vi "PH_BL-Master.PC _getVacPressuress.vi"(0 "i ref in":refnum<vi>, 2 "Channel Name":string="N/A", 3 "Value":dbl, 5 "error in (no error)":errorcluster) -> (14 "i ref out":refnum<vi>, 19 "error out":errorcluster)   [LabVIEW 2014, in "PH_BL-Master.lvlib"]
doc: "This VI writes the incoming information to own attributes."
uses:
  PH_BL-Master.lvlib
panel:
  in  "no link":bool
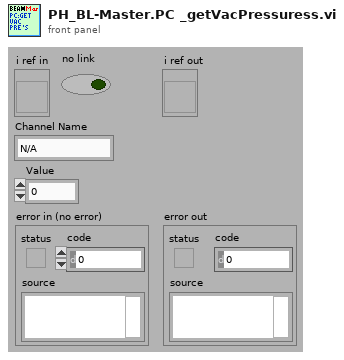
[diagram p1: front panel]
types:
  T1 = typedef "PH_BL-Master.lvlib/PH_BL-Master.i attribute.ctl" = cluster{"Remote controlled":bool, "Boolean Condition Service Subscriber":refnum<vi>[], "Picture Condition Service Subscriber":refnum<vi>[], "R2S":cluster{"GUI Ref":refnum<vi>, "State":bool}, "Vacua":cluster{"GUI Ref":refnum<vi>, "Limit":dbl, "Curr Value":dbl, "in range":bool}[], "O2 Inspection":cluster{"GUI Ref":refnum<vi>, "Concentration":dbl, "State":T2}[], "Boolean Status Service Subscriber":cluster{"GUI Ref":refnum<vi>, "Status":T2, "no Link?":bool, "Status Subscriber Class":T3}[], "Picture Status Service Subscriber":cluster{"GUI Ref":refnum<vi>, "Status":T2, "no Link?":bool, "Status Subscriber Class":T3}[], "6P 4Q Service Subscriber":cluster{"GUI Ref":refnum<vi>, "Selector":T4, "no Link?":bool}[], "Index of latest 6P 4Q changing Instance":i32, "Index of latest Picture Status changing Instance":i32, "Index of latest Boolean Status changing Instance":i32, "Vision ID on same Node":string, "Start Phase over?":bool, "GUI Ref Delete":refnum<vi>}
  T2 = typedef "PH_StatusHandler.lvlib/PH_StatusHandler.Status.ctl" = i16
  T3 = typedef "PH_BL-Master.lvlib/PH_BL-Master.Status Subscriber Class.ctl" = enum16{"unknown", "Switch", "BB", "6P Switch", "Switch GUI", "Switch and 6P State", "Force Sensor"}
  T4 = typedef "PH_4_Pos_Selector.lvlib/PH_4_Pos_Selector.Position Selector.ctl" = u16
  T5 = cluster{"GUI Ref":refnum<vi>, "Limit":dbl, "Curr Value":dbl, "in range":bool}[]
  T6 = cluster{"GUI Ref":refnum<vi>, "Limit":dbl, "Curr Value":dbl, "in range":bool}
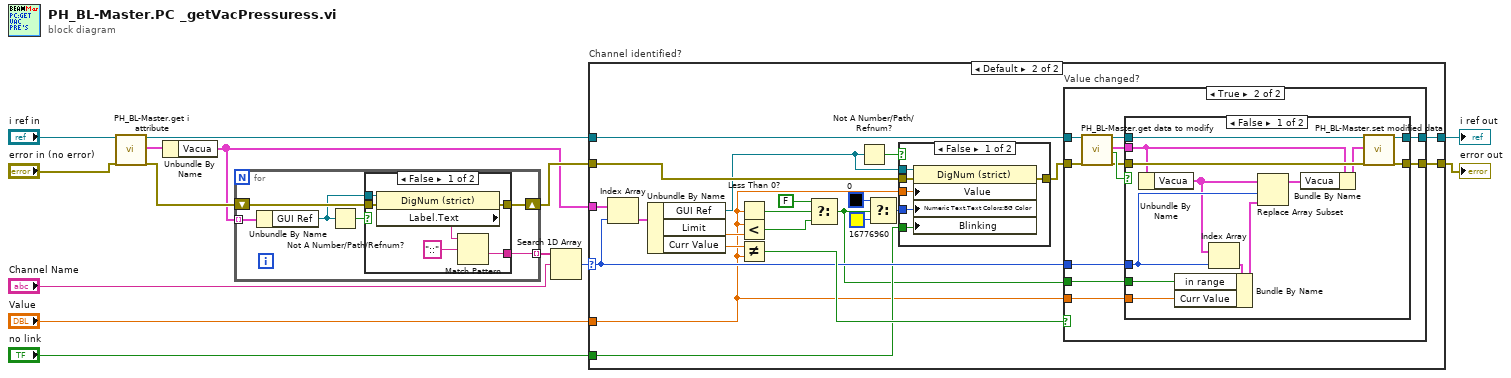
[diagram p0: block diagram]
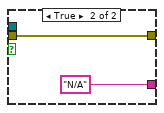
[diagram p2: hidden frame]
diagram:
  n1 = call "PH_BL-Master.get i attribute.vi"("i ref in"="i ref in", "error in (no error)"="error in (no error)") -> ("i ref out"=w9:refnum<vi>, "i attribute"=w8:T1, "error out"=w5:errorcluster)  [unwired: 15 in]
  n2 = Unbundle By Name(w8) -> ("Vacua"=w2:T5)
  n3 = for {
    tunnel: w2 -> [w20] mode=indexing
    tunnel: [w19] -> w3 mode=indexing
    shift-right: [w18] -> w4
    shift-left: w5 -> [w17]
    n4 = Unbundle By Name(w20) -> ("GUI Ref"=w15:refnum<vi>)
    n5 = Not A Number/Path/Refnum?(number/path/refnum=w15) -> (NaN/Path/Refnum?=w16:bool)
    n6 = case shown="False" w16 {
      tunnel: w15 -> [w26 _]
      tunnel: [w23 "N/A" ("Label.Text")] -> w19
      tunnel: [w22 w28] -> w18
      tunnel: w17 -> [w21 w28]
      frame False {
        n7 = property class="DigNum (strict)"(reference=w26, error in=w21) -> (error out=w22:errorcluster, "Label.Text"=w25:string)  [unwired: 1 out]
        n8 = Match Pattern(string=w25, regular expression="::") -> (after substring=w23:string)  [unwired: 1 in, 3 out]
      }
      frame True {
      }
    }
  }
  n9 = Search 1D Array(1D array=w3, element="Channel Name") -> (index of element=w7:i32)  [unwired: 1 in]
  n10 = case "Channel identified?" shown="Default" w7 {
    selector: w7 -> [_ w44]
    tunnel: [w29 w52] -> w14
    tunnel: [w30 w51] -> w13
    tunnel: "Value" -> [_ w32]
    tunnel: w4 -> [w29 w43]
    tunnel: w9 -> [w30 w50]
    tunnel: w2 -> [_ w49]
    tunnel: "no link" -> [_ w41]
    frame -1 {
    }
    frame Default {
      n11 = Index Array(array=w49, index=w44) -> (element=w48:T6)
      n12 = Unbundle By Name(w48) -> ("GUI Ref"=w31:refnum<vi>, "Limit"=w34:dbl, "Curr Value"=w47:dbl)
      n13 = Less Than 0?(x=w32) -> (x < 0?=w38:bool)
      n14 = Less?(x=w32, y=w34) -> (x < y?=w36:bool)
      n15 = Not Equal?(x=w47, y=w32) -> (x != y?=w46:bool)
      n16 = Select(t=FALSE, s=w38, f=w36) -> (s? t:f=w33:bool)
      n17 = Not A Number/Path/Refnum?(number/path/refnum=w31) -> (NaN/Path/Refnum?=w45:bool)
      n18 = Select(t=u32 0 ("Color Box"), s=w33, f=u32 16776960 ("Color Box")) -> (s? t:f=w35:u32)
      n19 = case shown="False" w45 {
        tunnel: w31 -> [w58 _]
        tunnel: w43 -> [w57 w59]
        tunnel: [w56 w59] -> w42
        tunnel: w32 -> [w55 _]
        tunnel: w35 -> [w54 _]
        tunnel: w41 -> [w53 _]
        frame False {
          n20 = property class="DigNum (strict)"(reference=w58, error in=w57, "Value"=w55, "Numeric Text.Text Colors:BG Color"=w54, "Blinking"=w53) -> (error out=w56:errorcluster)  [unwired: 1 out]
        }
        frame True {
        }
      }
      n21 = case "Value changed?" shown="True" w46 {
        tunnel: [w60 w70] -> w52
        tunnel: [w61 w68] -> w51
        tunnel: w42 -> [w60 w66]
        tunnel: w50 -> [w61 w65]
        tunnel: w44 -> [_ w64]
        tunnel: w32 -> [_ w63]
        tunnel: w33 -> [_ w62]
        frame False {
        }
        frame True {
          n22 = call "PH_BL-Master.get data to modify.vi"("i ref in"=w65, "error in (no error)"=w66) -> ("i ref out"=w67:refnum<vi>, "i attribute"=w71:T1, "timed out"=w72:bool, "error out"=w69:errorcluster)  [unwired: 14 in]
          n23 = case shown="False" w72 {
            tunnel: w67 -> [w85 w87]
            tunnel: [w84 w87] -> w68
            tunnel: w69 -> [w82 w86]
            tunnel: [w83 w86] -> w70
            tunnel: w71 -> [w80 _]
            tunnel: w63 -> [w79 _]
            tunnel: w64 -> [w78 _]
            tunnel: w62 -> [w73 _]
            frame False {
              n24 = Unbundle By Name(w80) -> ("Vacua"=w76:T5)
              n25 = Index Array(array=w76, index=w78) -> (element=w75:T6)
              n26 = Bundle By Name(cluster=w75, "in range"=w73, "Curr Value"=w79) -> (w74:T6)
              n27 = Replace Array Subset(array=w76, new element=w74, index=w78) -> (w77:T5)
              n28 = Bundle By Name(cluster=w80, "Vacua"=w77) -> (w81:T1)
              n29 = call "PH_BL-Master.set modified data.vi"("i ref in"=w85, "i attribute"=w81, "error in (no error)"=w82) -> ("i ref out"=w84:refnum<vi>, "error out"=w83:errorcluster)  [unwired: 15 in]
            }
            frame True {
            }
          }
        }
      }
    }
  }
  "error out" <- w14
  "i ref out" <- w13
